vi "Kiwi_Angle_Cal.vi"(6 "Radians?":bool, 8 "Angle C":dbl, 9 "Angle B":dbl, 10 "Angle A":dbl, 11 "MotorDevRefIn":T1={"Motor A"={"DeviceStatus"={"status"=FALSE, "code"=0, "source"=""}, "Type"=enum."PWM", "PWM"={"PWM Channel"=enum."Invalid", "DeadBand"={"Name"="", "maxPositivePwm"=0, "minPositivePwm"=0, "centerPwm"=0, "maxNegativePwm"=0, "minNegativePwm"=0, "angularRange"=0}}, "CAN"={"Device Number"=0, "Control Mode"=enum."Percent VBus", "Semaphore"=refnum, "Max Vout"=12.0, "TalonSRX Control Mode"=enum."Percent VBus"}, "Invert"=FALSE}, "Motor B"={"DeviceStatus"={"status"=FALSE, "code"=0, "source"=""}, "Type"=enum."PWM", "PWM"={"PWM Channel"=enum."Invalid", "DeadBand"={"Name"="", "maxPositivePwm"=0, "minPositivePwm"=0, "centerPwm"=0, "maxNegativePwm"=0, "minNegativePwm"=0, "angularRange"=0}}, "CAN"={"Device Number"=0, "Control Mode"=enum."Percent VBus", "Semaphore"=refnum, "Max Vout"=12.0, "TalonSRX Control Mode"=enum."Percent VBus"}, "Invert"=FALSE}, "Motor C"={"DeviceStatus"={"status"=FALSE, "code"=0, "source"=""}, "Type"=enum."PWM", "PWM"={"PWM Channel"=enum."Invalid", "DeadBand"={"Name"="", "maxPositivePwm"=0, "minPositivePwm"=0, "centerPwm"=0, "maxNegativePwm"=0, "minNegativePwm"=0, "angularRange"=0}}, "CAN"={"Device Number"=0, "Control Mode"=enum."Percent VBus", "Semaphore"=refnum, "Max Vout"=12.0, "TalonSRX Control Mode"=enum."Percent VBus"}, "Invert"=FALSE}, "Config Consts"={"Arx"=0.0, "Ay"=0.0, "Brx"=0.0, "By"=0.0, "Cr"=0.0, "Cy"=0.0, "Cx"=0.0}, "status"={"status"=FALSE, "code"=0, "source"=""}, "Angles"={"Angle A"=60.0, "Angle B"=60.0, "Angle C"=60.0, "Radians?"=FALSE}, "MotorVals"={"MotorA"=0.0, "MotorB"=0.0, "MotorC"=0.0}}) -> (0 "error out":errorcluster, 2 "Config Consts":T9, 3 "MotorDevRefOut":T1={"Motor A"={"DeviceStatus"={"status"=FALSE, "code"=0, "source"=""}, "Type"=enum."PWM", "PWM"={"PWM Channel"=enum."Invalid", "DeadBand"={"Name"="", "maxPositivePwm"=0, "minPositivePwm"=0, "centerPwm"=0, "maxNegativePwm"=0, "minNegativePwm"=0, "angularRange"=0}}, "CAN"={"Device Number"=0, "Control Mode"=enum."Percent VBus", "Semaphore"=refnum, "Max Vout"=12.0, "TalonSRX Control Mode"=enum."Percent VBus"}, "Invert"=FALSE}, "Motor B"={"DeviceStatus"={"status"=FALSE, "code"=0, "source"=""}, "Type"=enum."PWM", "PWM"={"PWM Channel"=enum."Invalid", "DeadBand"={"Name"="", "maxPositivePwm"=0, "minPositivePwm"=0, "centerPwm"=0, "maxNegativePwm"=0, "minNegativePwm"=0, "angularRange"=0}}, "CAN"={"Device Number"=0, "Control Mode"=enum."Percent VBus", "Semaphore"=refnum, "Max Vout"=12.0, "TalonSRX Control Mode"=enum."Percent VBus"}, "Invert"=FALSE}, "Motor C"={"DeviceStatus"={"status"=FALSE, "code"=0, "source"=""}, "Type"=enum."PWM", "PWM"={"PWM Channel"=enum."Invalid", "DeadBand"={"Name"="", "maxPositivePwm"=0, "minPositivePwm"=0, "centerPwm"=0, "maxNegativePwm"=0, "minNegativePwm"=0, "angularRange"=0}}, "CAN"={"Device Number"=0, "Control Mode"=enum."Percent VBus", "Semaphore"=refnum, "Max Vout"=12.0, "TalonSRX Control Mode"=enum."Percent VBus"}, "Invert"=FALSE}, "Config Consts"={"Arx"=0.0, "Ay"=0.0, "Brx"=0.0, "By"=0.0, "Cr"=0.0, "Cy"=0.0, "Cx"=0.0}, "status"={"status"=FALSE, "code"=0, "source"=""}, "Angles"={"Angle A"=60.0, "Angle B"=60.0, "Angle C"=60.0, "Radians?"=FALSE}, "MotorVals"={"MotorA"=0.0, "MotorB"=0.0, "MotorC"=0.0}})   [LabVIEW 2015]
uses:
  <userlib>/836-Library/Drive/kiwi/support/Kiwi_Cal_Constants.ctl
  <userlib>/836-Library/Drive/kiwi/support/Kiwi_Dev_Ref.ctl
  <vilib>/Rock Robotics/WPI/MotorControl/WPI_MotorControlDeviceRef.ctl
  <vilib>/Rock Robotics/WPI/MotorControl/WPI_MotorControlType.ctl
  <vilib>/Rock Robotics/SystemInterfaces/DIO/FPGA_DIOPWMChannel.ctl
  <vilib>/Rock Robotics/WPI/PWM/WPI_PWMDeadband.ctl
  <vilib>/Rock Robotics/WPI/CAN/Jaguar/SubVIs/WPI_CANJaguar_ControlMode.ctl
  <vilib>/Rock Robotics/WPI/CAN/TalonSRX/WPI_CANTalonSRX_APIControlMode.ctl
  <userlib>/836-Library/Drive/kiwi/support/Kiwi_Angles.ctl
  <vilib>/Utility/error.llb/Error Cluster From Error Code.vi
  <vilib>/ErrorRing/Error Ring.xnode
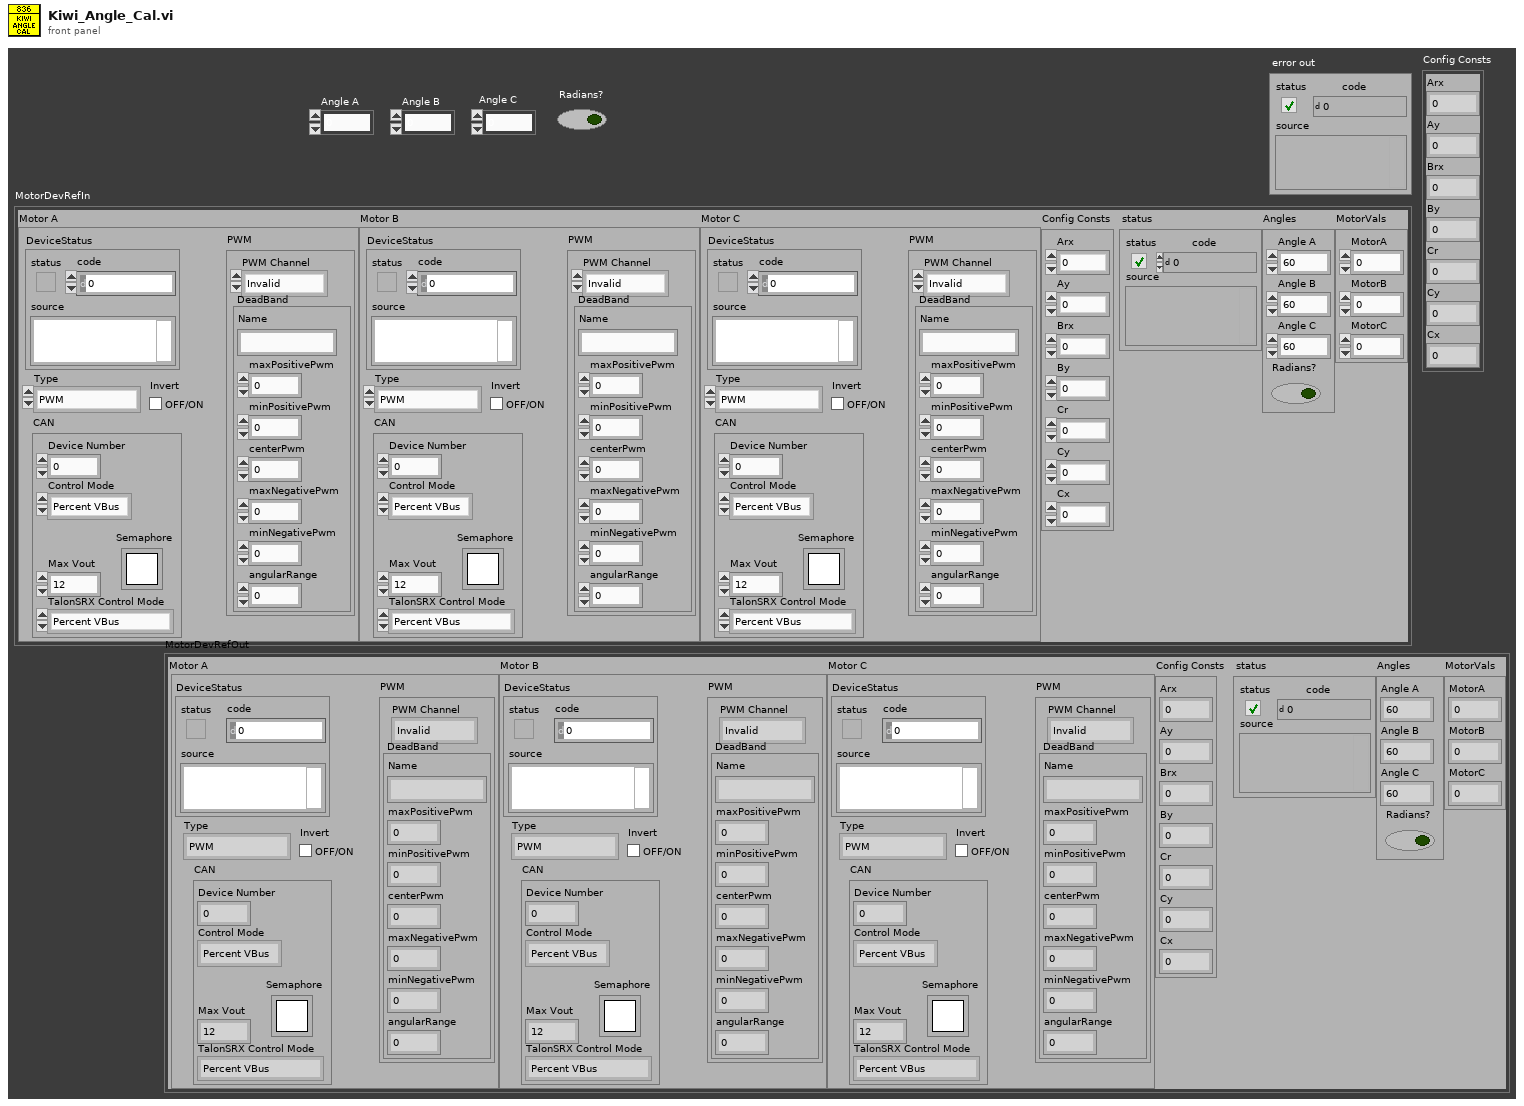
[diagram p1: front panel]
types:
  T1 = typedef "Kiwi_Dev_Ref.ctl" = cluster{"Motor A":T2, "Motor B":T2, "Motor C":T2, "Config Consts":T9, "status":errorcluster, "Angles":T10, "MotorVals":cluster{"MotorA":dbl, "MotorB":dbl, "MotorC":dbl}}
  T2 = typedef "WPI_MotorControlDeviceRef.ctl" = cluster{"DeviceStatus":errorcluster, "Type":T3, "PWM":cluster{"PWM Channel":T4, "DeadBand":T5}, "CAN":cluster{"Device Number":u8, "Control Mode":T6, "Semaphore":T7, "Max Vout":dbl, "TalonSRX Control Mode":T8}, "Invert":bool}
  T3 = typedef "WPI_MotorControlType.ctl" = enum16{"PWM", "CAN", "CANTalonSRX"}
  T4 = typedef "FPGA_DIOPWMChannel.ctl" = enum8{"PWM 0", "PWM 1", "PWM 2", "PWM 3", "PWM 4", "PWM 5", "PWM 6", "PWM 7", "PWM 8", "PWM 9", "PWM MXP 0", "PWM MXP 1", "PWM MXP 2", "PWM MXP 3", "PWM MXP 4", "PWM MXP 5", "PWM MXP 6", "PWM MXP 7", "PWM MXP 8", "PWM MXP 9", "Invalid"}
  T5 = typedef "WPI_PWMDeadband.ctl" = cluster{"Name":string, "maxPositivePwm":i32, "minPositivePwm":i32, "centerPwm":i32, "maxNegativePwm":i32, "minNegativePwm":i32, "angularRange":u16}
  T6 = typedef "WPI_CANJaguar_ControlMode.ctl" = enum8{"Percent VBus", "Current", "Speed", "Position", "Voltage"}
  T7 = typedef "Semaphore RefNum" = refnum<k1>
  T8 = typedef "WPI_CANTalonSRX_APIControlMode.ctl" = enum8{"Percent VBus", "Speed", "Position", "Slave", "Unchanged / Invalid", "Voltage Compensation", "Current", "Motion Profile"}
  T9 = typedef "Kiwi_Cal_Constants.ctl" = cluster{"Arx":dbl, "Ay":dbl, "Brx":dbl, "By":dbl, "Cr":dbl, "Cy":dbl, "Cx":dbl}
  T10 = typedef "Kiwi_Angles.ctl" = cluster{"Angle A":dbl, "Angle B":dbl, "Angle C":dbl, "Radians?":bool}
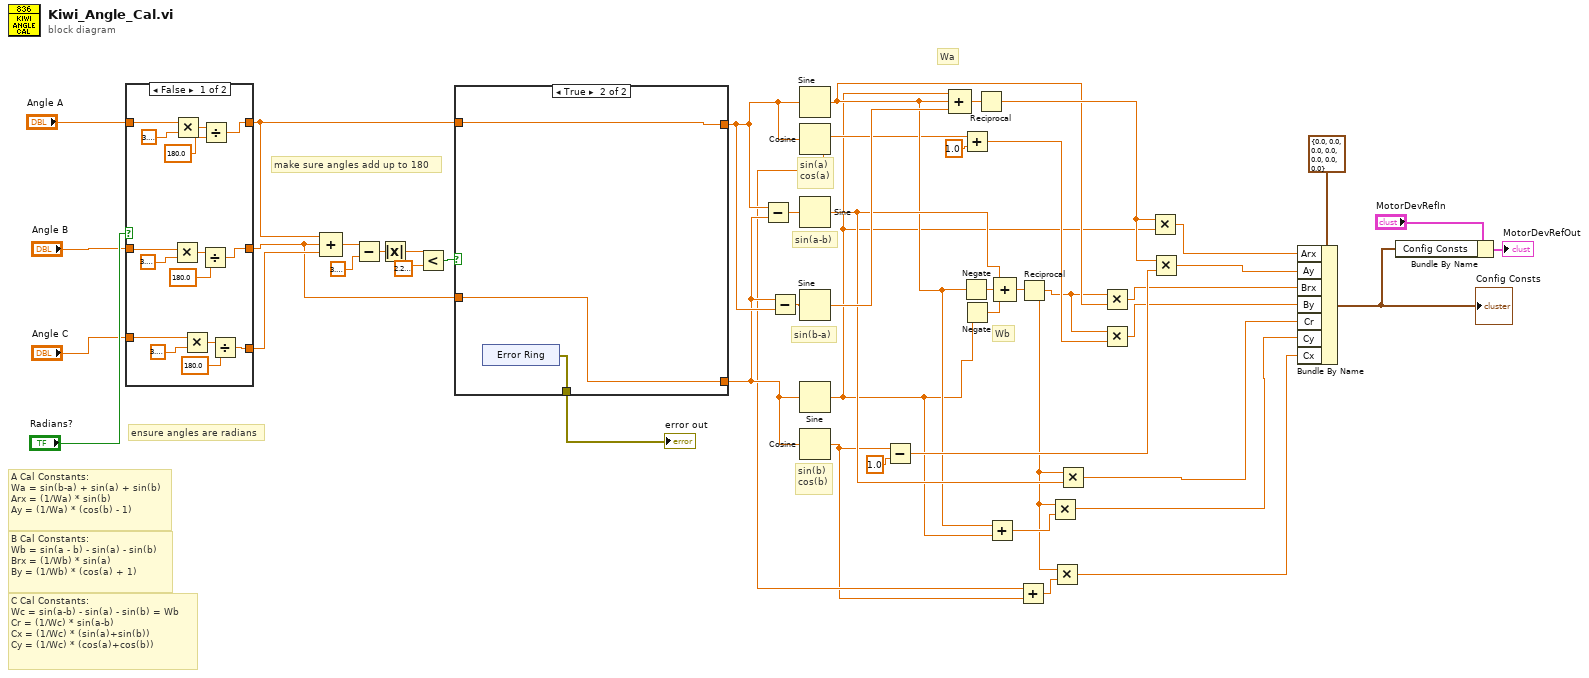
[diagram p0: block diagram]
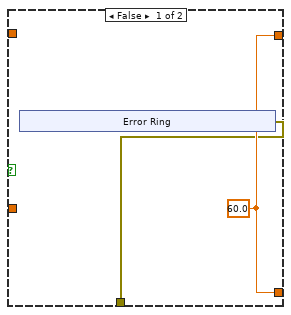
[diagram p2: hidden frame]
diagram:
  # "Wb"
  # "Wa"
  # "sin(b)\ncos(b)"
  # "sin(a)\ncos(a)"
  # "sin(a-b)"
  # "sin(b-a)"
  # "make sure angles add up to 180"
  # "ensure angles are radians"
  # "B Cal Constants:\nWb = sin(a - b) - sin(a) - sin(b)\nBrx = (1/Wb) * sin(a)\nBy = (1/Wb) * (cos(a) + 1)"
  # "A Cal Constants:\nWa = sin(b-a) + sin(a) + sin(b)\nArx = (1/Wa) * sin(b)\nAy = (1/Wa) * (cos(b) - 1)"
  # "C Cal Constants:\nWc = sin(a-b) - sin(a) - sin(b) = Wb\nCr = (1/Wc) * sin(a-b)\nCx = (1/Wc) * (sin(a)+sin(b))\nCy = (1/Wc) * (cos(a)+cos(b))"
  n1 = case shown="False" "Radians?" {
    tunnel: "Angle C" -> [w55 w63]
    tunnel: "Angle B" -> [w62 w64]
    tunnel: "Angle A" -> [w51 w65]
    tunnel: [w50 w65] -> w37
    tunnel: [w59 w64] -> w35
    tunnel: [w54 w63] -> w36
    frame False {
      n2 = Multiply(x=w62, y=3.141592653589793) -> (x*y=w60:dbl)
      n3 = Multiply(x=w51, y=3.141592653589793) -> (x*y=w53:dbl)
      n4 = Multiply(x=w55, y=3.141592653589793) -> (x*y=w57:dbl)
      n5 = Divide(x=w60, y=180.0) -> (x/y=w59:dbl)
      n6 = Divide(x=w53, y=180.0) -> (x/y=w50:dbl)
      n7 = Divide(x=w57, y=180.0) -> (x/y=w54:dbl)
    }
    frame True {
    }
  }
  n8 = Compound Arithmetic op=ADD(w37, w35, w36) -> (w42:dbl)
  n9 = Subtract(x=w42, y=3.141592653589793) -> (x-y=w40:dbl)
  n10 = Absolute Value(x=w40) -> (abs(x)=w39:dbl)
  n11 = Less?(x=w39, y=2.220446049250313e-16) -> (x < y?=w38:bool)
  n12 = case shown="True" w38 {
    tunnel: [w67 w75] -> w32
    tunnel: w37 -> [_ w75]
    tunnel: w35 -> [_ w74]
    tunnel: [w67 w74] -> w31
    tunnel: [w66 w73] -> w8
    frame False {
      w67 = 60.0
      n13 = xnode "Error Ring"() -> ("error out"=w66:errorcluster)
    }
    frame True {
      n14 = xnode "Error Ring"() -> ("error out"=w73:errorcluster)
    }
  }
  "error out" <- w8
  n15 = Subtract(x=w32, y=w31) -> (x-y=w33:dbl)
  n16 = Subtract(x=w31, y=w32) -> (x-y=w34:dbl)
  n17 = Sine(x=w32) -> (sin(x)=w16:dbl)
  n18 = Cosine(x=w32) -> (cos(x)=w11:dbl)
  n19 = Sine(x=w33) -> (sin(x)=w17:dbl)
  n20 = Sine(x=w34) -> (sin(x)=w30:dbl)
  n21 = Sine(x=w31) -> (sin(x)=w4:dbl)
  n22 = Cosine(x=w31) -> (cos(x)=w10:dbl)
  n23 = Subtract(x=w10, y=1.0) -> (x-y=w24:dbl)
  n24 = Compound Arithmetic op=ADD(w4, w16, w30) -> (w29:dbl)
  n25 = Negate(x=w16) -> (-x=w22:dbl)
  n26 = Add(x=w11, y=1.0) -> (x+y=w19:dbl)
  n27 = Negate(x=w4) -> (-x=w21:dbl)
  n28 = Reciprocal(x=w29) -> (1/x=w26:dbl)
  n29 = Add(x=w16, y=w4) -> (x+y=w15:dbl)
  n30 = Compound Arithmetic op=ADD(w17, w22, w21) -> (w23:dbl)
  n31 = Add(x=w11, y=w10) -> (x+y=w12:dbl)
  n32 = Reciprocal(x=w23) -> (1/x=w13:dbl)
  n33 = Multiply(x=w13, y=w15) -> (x*y=w14:dbl)
  n34 = Multiply(x=w13, y=w12) -> (x*y=w9:dbl)
  n35 = Multiply(x=w13, y=w17) -> (x*y=w1:dbl)
  n36 = Multiply(x=w13, y=w16) -> (x*y=w2:dbl)
  n37 = Multiply(x=w13, y=w19) -> (x*y=w18:dbl)
  n38 = Multiply(x=w26, y=w4) -> (x*y=w3:dbl)
  n39 = Multiply(x=w26, y=w24) -> (x*y=w27:dbl)
  n40 = Bundle By Name(cluster=T9 {"Arx"=0.0, "Ay"=0.0, "Brx"=0.0, "By"=0.0, "Cr"=0.0, "Cy"=0.0, "Cx"=0.0} ("Config Consts 2"), "Arx"=w3, "Ay"=w27, "Brx"=w2, "By"=w18, "Cr"=w1, "Cy"=w14, "Cx"=w9) -> (w6:T9)
  "Config Consts" <- w6
  n41 = Bundle By Name(cluster="MotorDevRefIn", "Config Consts"=w6) -> (→"MotorDevRefOut":T1)
